vi "raptor_start.vi"(8 "error in (no error)":errorcluster) -> (0 "error out":errorcluster)   [LabVIEW 2016]
doc: "Raptor: Continues processing. Only needed if this was previously stopped using raptor_stop."
uses:
  typedef/raptor_message.ctl
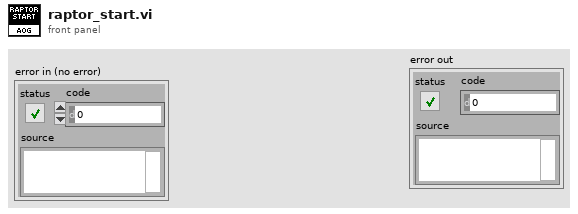
[diagram p1: front panel]
types:
  T1 = typedef "raptor_message.ctl" = cluster{"Message":enum16{"start", "stop", "initialise", "shutdown", "end scan", "new scan", "set depth"}, "Data":variant}
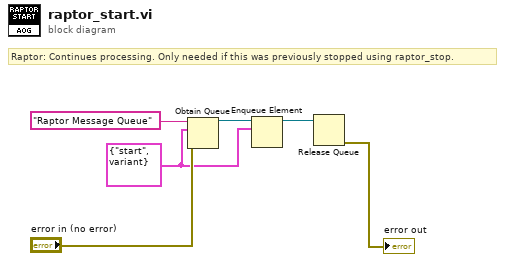
[diagram p0: block diagram]
diagram:
  w3 = T1 {"Message"=enum."start", "Data"=variant} ("Cluster")
  # "Raptor: Continues processing. Only needed if this was previously stopped using raptor_stop."
  n1 = Obtain Queue(name (unnamed)="Raptor Message Queue", element data type=w3, error in (no error)="error in (no error)") -> (queue out=w4:refnum<queue>)  [unwired: 2 in, 2 out]
  n2 = Enqueue Element(queue=w4, element=w3) -> (queue out=w2:refnum<queue>)  [unwired: 2 in, 2 out]
  n3 = Release Queue(queue=w2) -> (error out=→"error out":errorcluster)  [unwired: 2 in, 2 out]
